vi "Scope.vi"(8 "REF_Y":waveform(dbl)[](array[waveform]), 9 "REF_X":waveform(dbl)[](array[waveform]), 10 "AI":waveform(dbl)[](array[waveform]), 11 "AO":waveform(dbl)[](array[waveform])) -> ()   [LabVIEW 2019, in "Instrument.Lockin.lvlib" / "Instrument.DAQ.lvclass"]
uses:
  Instrument.DAQ.lvclass
panel:
  out "Waveform Graph":waveform(dbl)[](graph)
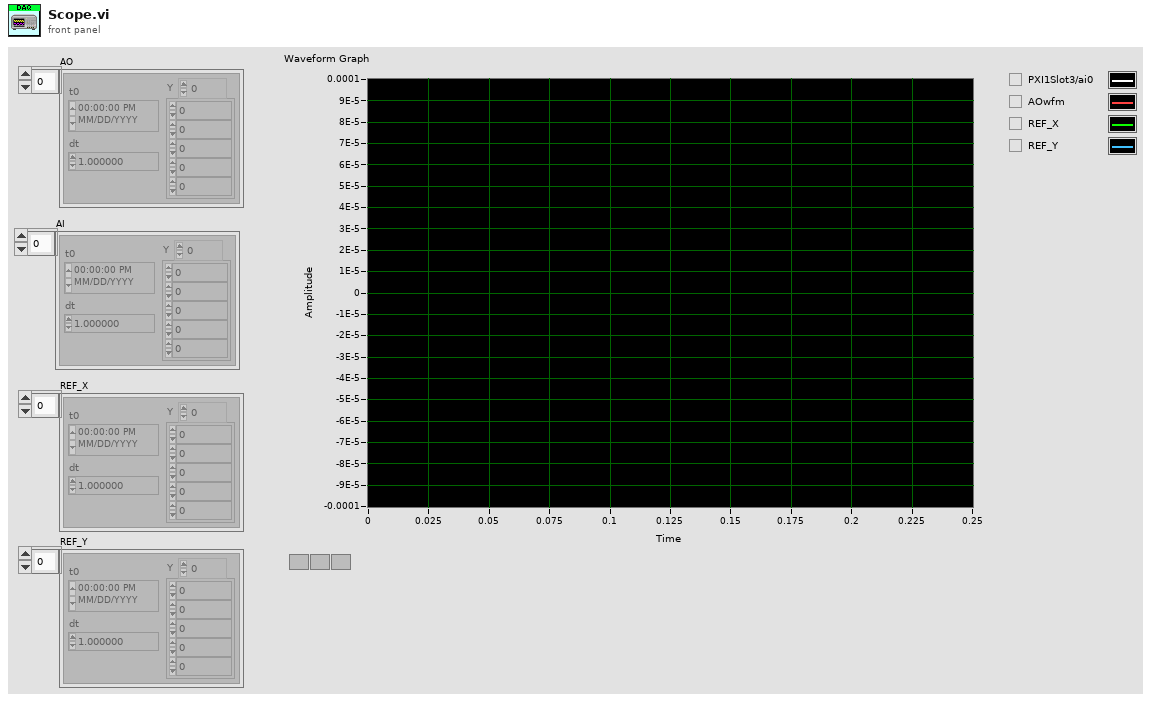
[diagram p1: front panel]
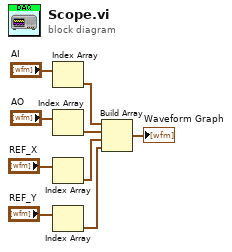
[diagram p0: block diagram]
diagram:
  n1 = Index Array(array="AI") -> (element=w7:waveform(dbl))  [unwired: 1 in]
  n2 = Index Array(array="AO") -> (element=w6:waveform(dbl))  [unwired: 1 in]
  n3 = Index Array(array="REF_X") -> (element=w9:waveform(dbl))  [unwired: 1 in]
  n4 = Index Array(array="REF_Y") -> (element=w8:waveform(dbl))  [unwired: 1 in]
  n5 = Build Array(w7, w6, w9, w8) -> (→"Waveform Graph":waveform(dbl)[])
